vi "Server UI.vi"(8 "error in (no error)":errorcluster, 11 "Chat Server in":refnum<class "Chat Server.lvclass">) -> (0 "error out":errorcluster, 3 "Chat Server out":refnum<class "Chat Server.lvclass">)   [LabVIEW 2020, in "Chat Server.lvclass"]
uses:
  Chat Server.lvclass
  lv-stream/stream/Connection/Connection.lvclass
  lv-stream/stream/Stream/Stream.lvclass
panel:
  out "Stop":bool
  out "Last Message":string
  out "Connected Clients":i32
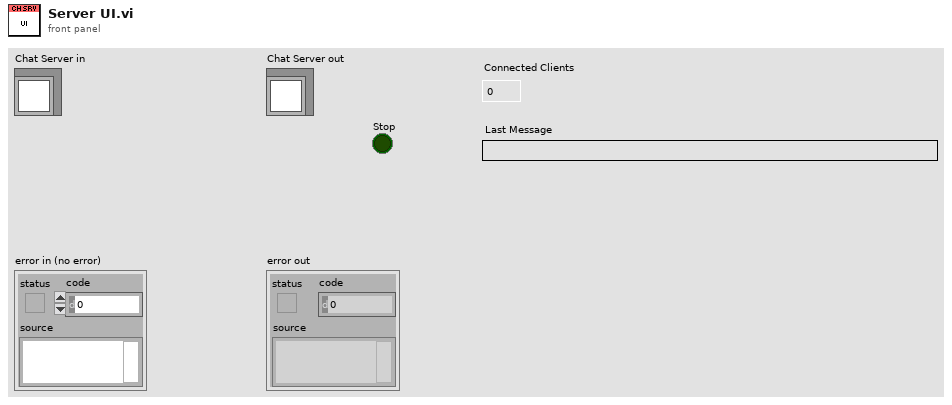
[diagram p1: front panel]
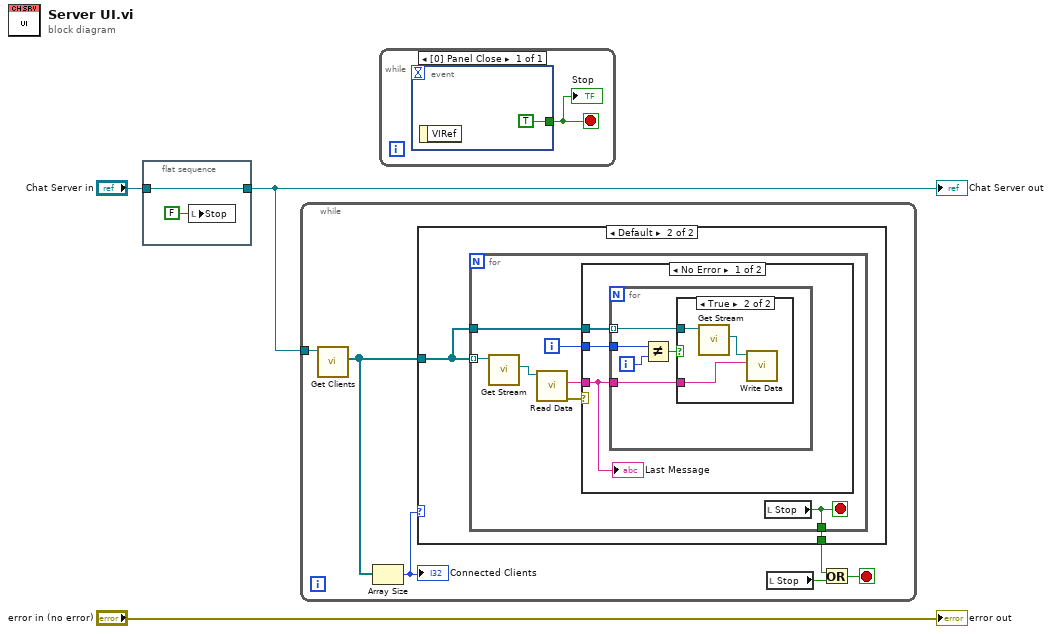
[diagram p0: block diagram]
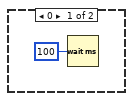
[diagram p2: hidden frame]
diagram:
  n1 = flat-sequence {
    tunnel: "Chat Server in" -> [w5]
    tunnel: [w5] -> w1
    frame #0 {
      n2 = local write "Stop"(FALSE ("Stop")) -> ()
    }
  }
  n3 = while {
    tunnel: w1 -> [w11]
    stop <- w9 stop-if-true
    n4 = call "Get Clients.vi"("Chat Server in"=w11) -> ("Connections"=w7:refnum<class "Connection.lvclass">[])  [unwired: 8 in, 2 out]
    n5 = Array Size(array=w7) -> (size(s)=w6:i32)
    "Connected Clients" <- w6
    n6 = case shown="Default" w6 {
      tunnel: [_ w14] -> w10
      tunnel: w7 -> [_ w13]
      frame 0 {
        n7 = Wait (ms)(milliseconds to wait=u32 100) -> ()  [unwired: 1 out]
      }
      frame Default {
        n8 = for {
          tunnel: w13 -> [w21] mode=indexing
          tunnel: w13 -> [w15]
          tunnel: [w19] -> w14
          i -> [w16]
          stop <- w19 stop-if-true
          n9 = call-dynamic "Get Stream.vi"("Connection in"=w21) -> ("Stream"=w20:refnum<class "Stream.lvclass">)  [unwired: 8 in, 2 out]
          n10 = call-dynamic "Read Data.vi"("Stream in"=w20) -> ("error out"=w18:errorcluster, "Data"=w17:string)  [unwired: 8 in, 1 out]
          n11 = case shown="No Error" w18 {
            tunnel: w17 -> [w22 _]
            tunnel: w16 -> [w23 _]
            tunnel: w15 -> [w24 _]
            frame No Error {
              n12 = for {
                tunnel: w24 -> [w26] mode=indexing
                tunnel: w23 -> [w29]
                tunnel: w22 -> [w25]
                i -> [w28]
                n13 = Not Equal?(x=w29, y=w28) -> (x != y?=w27:bool)
                n14 = case shown="True" w27 {
                  tunnel: w26 -> [_ w32]
                  tunnel: w25 -> [_ w30]
                  frame False {
                  }
                  frame True {
                    n15 = call-dynamic "Get Stream.vi"("Connection in"=w32) -> ("Stream"=w31:refnum<class "Stream.lvclass">)  [unwired: 8 in, 2 out]
                    n16 = call-dynamic "Write Data.vi"("Data"=w30, "Stream in"=w31) -> ()  [unwired: 8 in, 2 out]
                  }
                }
              }
              "Last Message" <- w22
            }
            frame Error {
            }
          }
          n17 = local read "Stop"() -> (w19:bool)
        }
      }
    }
    n18 = local read "Stop"() -> (w8:bool)
    n19 = Or(x=w10, y=w8) -> (x .or. y?=w9:bool)
  }
  n20 = while {
    stop <- w33 stop-if-true
    n21 = event shown="[0] Panel Close" {
      selector: _ -> [_]
      dyn-events: _ -> [_]
      timeout: _ -> [_]
      tunnel: [TRUE] -> w33
      event Panel Close {
        n22 = event-data() -> ()  [unwired: 1 in, 1 out]
      }
    }
    "Stop" <- w33
  }
  "error out" <- "error in (no error)"
  "Chat Server out" <- w1
